vi "Knob6.vi"() -> ()   [LabVIEW 2017]
panel:
  out "Thermometer":dbl(slide) scale=0.0..100.0
  in  "Knob":i8(knob) scale=0.0..2.0
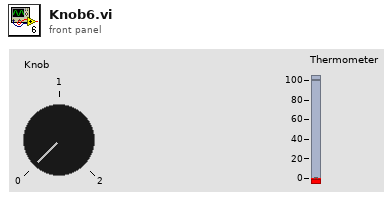
[diagram p1: front panel]
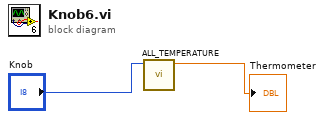
[diagram p0: block diagram]
diagram:
  n1 = call "ALL_TEMPERATURE.vi"("Numeric"="Knob") -> ("F"=→"Thermometer":dbl)  [unwired: 10 in]
